vi "RSZVB Calibration Auto Assignment Definition.vi"(0 "VISA resource name":refnum<visa-resource-name>, 1 "Analyzer Port 2 (0)":i32, 2 "Analyzer Port 4 (0)":i32, 3 "Cal Unit Port 2 (0)":i32, 5 "Channel (1)":i32=1, 7 "Assignment (1)":i32=1, 9 "Analyzer Port 1 (1)":i32=1, 10 "Cal Unit Port 4 (0)":i32, 11 "error in (no error)":errorcluster {"code" format="%.0x"}, 12 "Analyzer Port 3 (0)":i32, 13 "Cal Unit Port 1 (1)":i32=1, 14 "Cal Unit Port 3 (0)":i32) -> (4 "VISA resource name out":refnum<visa-resource-name>, 15 "error out":errorcluster {"code" format="%.0x"})   [LabVIEW 2011]
doc: "This VI defines a port assignment numbered <Assignment>. This command is particularly relevant for multiple port\nassignments.\n\nRemote-control command(s):\n[SENSe<Ch>:]CORRection:COLLect:AUTO:ASSignment<Asg>:DEFine <analyzer_port_no>,<cal_unit_port_no>{,<analyzer_port_no>,<cal_unit_port_no>}"
uses:
  _utility/RSZVB Global Data.vi
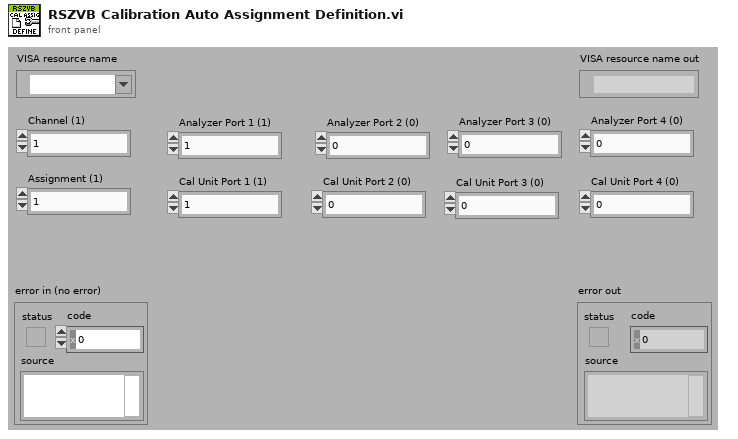
[diagram p1: front panel]
types:
  T1 = cluster{"Error Checking (T: On)":bool, "Installed Options":string[], "Data Valid?":bool, "Ports":i32, "Model":string[], "Option Checking (T: On)":bool}[]
  T2 = cluster{"Error Checking (T: On)":bool, "Installed Options":string[], "Data Valid?":bool, "Ports":i32, "Model":string[], "Option Checking (T: On)":bool}
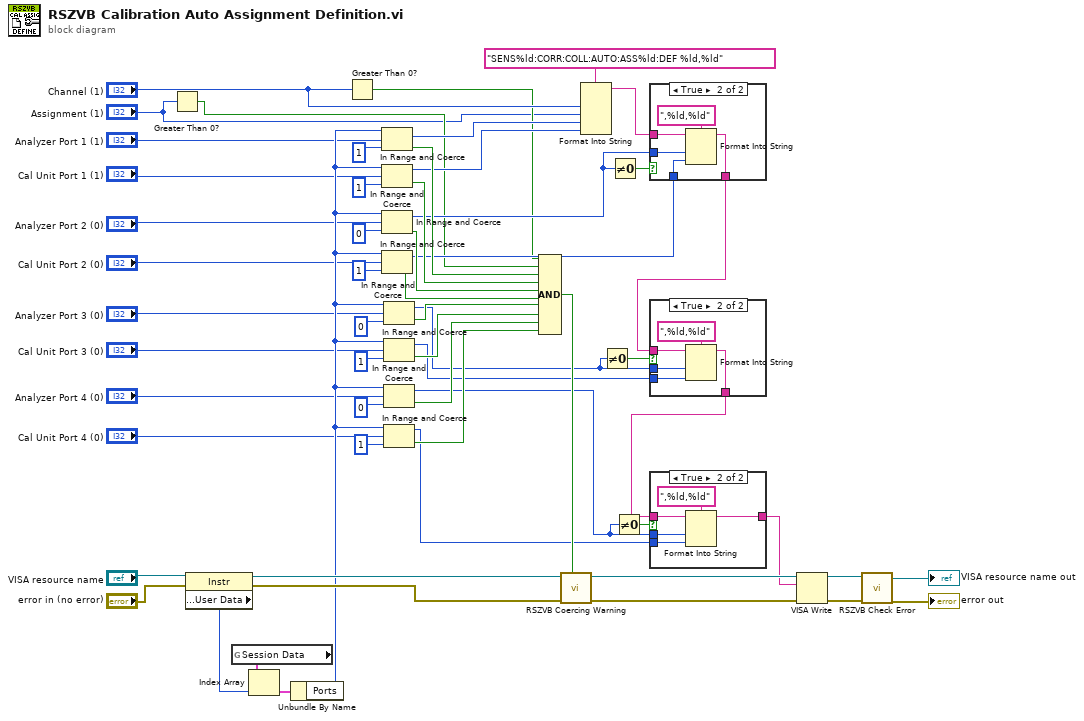
[diagram p0: block diagram]
diagram:
  n1 = Greater Than 0?(x="Assignment (1)") -> (x > 0?=w10:bool)
  n2 = property class="Instr"(reference="VISA resource name", error in="error in (no error)") -> (reference out=w51:refnum<visa-resource-name>, error out=w52:errorcluster, "General Settings:User Data"=w53:u32)
  n3 = global read "RSZVB Global Data.vi" "Session Data"() -> (w54:T1)
  n4 = Index Array(array=w54, index=w53) -> (element=w55:T2)
  n5 = Unbundle By Name(w55) -> ("Ports"=w28:i32)
  n6 = Greater Than 0?(x="Channel (1)") -> (x > 0?=w11:bool)
  n7 = In Range and Coerce(upper limit=w28, x="Analyzer Port 1 (1)", lower limit=1) -> (coerced(x)=w35:i32, In Range?=w47:bool)
  n8 = In Range and Coerce(upper limit=w28, x="Cal Unit Port 1 (1)", lower limit=1) -> (coerced(x)=w25:i32, In Range?=w46:bool)
  n9 = In Range and Coerce(upper limit=w28, x="Analyzer Port 2 (0)", lower limit=0) -> (coerced(x)=w24:i32, In Range?=w45:bool)
  n10 = In Range and Coerce(upper limit=w28, x="Cal Unit Port 2 (0)", lower limit=1) -> (coerced(x)=w23:i32, In Range?=w44:bool)
  n11 = In Range and Coerce(upper limit=w28, x="Analyzer Port 3 (0)", lower limit=0) -> (coerced(x)=w20:i32, In Range?=w33:bool)
  n12 = In Range and Coerce(upper limit=w28, x="Cal Unit Port 3 (0)", lower limit=1) -> (coerced(x)=w22:i32, In Range?=w32:bool)
  n13 = In Range and Coerce(upper limit=w28, x="Analyzer Port 4 (0)", lower limit=0) -> (coerced(x)=w19:i32, In Range?=w31:bool)
  n14 = In Range and Coerce(upper limit=w28, x="Cal Unit Port 4 (0)", lower limit=1) -> (coerced(x)=w21:i32, In Range?=w30:bool)
  n15 = Compound Arithmetic op=AND(w11, w10, w47, w46, w45, w44, w33, w32, w31, w30) -> (w56:bool)
  n16 = call "RSZVB Coercing Warning.vi"("In Range?"=w56, "error in (no error)"=w52, "VISA session"=w51) -> ("error out"=w57:errorcluster, "dup VISA session"=w58:refnum<visa-resource-name>)  [unwired: 7 in]
  n17 = Format Into String(format string="SENS%ld:CORR:COLL:AUTO:ASS%ld:DEF %ld,%ld", "Channel (1)", "Assignment (1)", w35, w25) -> (resulting string=w41:string)  [unwired: 2 in, 1 out]
  n18 = Not Equal To 0?(x=w20) -> (x != 0?=w40:bool)
  n19 = Not Equal To 0?(x=w24) -> (x != 0?=w42:bool)
  n20 = Not Equal To 0?(x=w19) -> (x != 0?=w38:bool)
  n21 = case shown="True" w42 {
    tunnel: w41 -> [w60 w65]
    tunnel: w24 -> [_ w63]
    tunnel: [w60 w62] -> w39
    tunnel: w23 -> [_ w61]
    frame False {
    }
    frame True {
      n22 = Format Into String(format string=",%ld,%ld", initial string=w65, w63, w61) -> (resulting string=w62:string)  [unwired: 1 in, 1 out]
    }
  }
  n23 = case shown="True" w40 {
    tunnel: w39 -> [w66 w71]
    tunnel: w20 -> [_ w69]
    tunnel: [w66 w68] -> w37
    tunnel: w22 -> [_ w67]
    frame False {
    }
    frame True {
      n24 = Format Into String(format string=",%ld,%ld", initial string=w71, w69, w67) -> (resulting string=w68:string)  [unwired: 1 in, 1 out]
    }
  }
  n25 = case shown="True" w38 {
    tunnel: w37 -> [w72 w77]
    tunnel: w19 -> [_ w75]
    tunnel: [w72 w74] -> w36
    tunnel: w21 -> [_ w73]
    frame False {
    }
    frame True {
      n26 = Format Into String(format string=",%ld,%ld", initial string=w77, w75, w73) -> (resulting string=w74:string)  [unwired: 1 in, 1 out]
    }
  }
  n27 = VISA Write(VISA resource name=w58, write buffer=w36, error in (no error)=w57) -> (VISA resource name out=w15:refnum<visa-resource-name>, error out=w16:errorcluster)  [unwired: 1 out]
  n28 = call "RSZVB Check Error.vi"("error in (no error)"=w16, "VISA session"=w15) -> ("error out"=→"error out":errorcluster, "dup VISA session"=→"VISA resource name out":refnum<visa-resource-name>)  [unwired: 8 in]
